vi "KN-OptionsToString.vi"(0 "Annulus IN":T2 {"End Angle" format="%.2f"; "Start Angle" format="%.2f"; "Center X" scale=0.0..1024.0}, 1 "Options IN":T5={"Search  Direction"=0, "Edge Options"={"Edge Polarity"=0, "Kernel Size"=13, "Width"=13, "Minimum Edge Strength"=52.0, "Interpolation Type"=enum."Bilinear Fixed", "Data Processing Method"=enum."Average"}} {"Search  Direction" items=["Outside to Inside", "Inside to Outside"]; "Edge Options"."Edge Polarity" items=["All Edges", "Rising Edges", "Falling Edges"]; "Edge Options"."Minimum Edge Strength" format="%.2f"; "Edge Options"."Width" step=2; "Edge Options"."Kernel Size" step=2}, 2 "Circle Fit Options":T1, 3 "(Color Threshold 1)":cluster{"Lower value":i32, "Upper value":i32}={"Lower value"=12, "Upper value"=253}) -> (14 "OptionsString Out":string=";1480.000;1115.000;378.000;757.000;0.000;0.000;0;1;3;3;10.000;4;0;1;1;1;1;65280;255;16776960;16711680;;3;10;3;23;255")   [LabVIEW 2015]
uses:
  <vilib>/vision/Measure.llb/Edge Options.ctl
  <vilib>/vision/Measure.llb/Edge Polarity.ctl
panel:
  out "Array":string[](array[string])
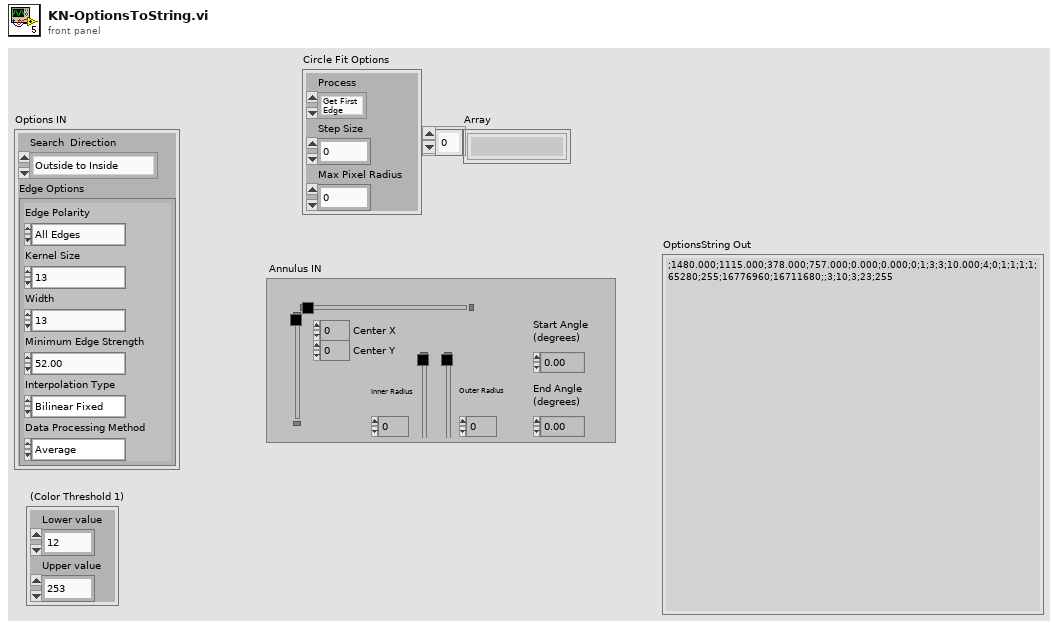
[diagram p1: front panel]
types:
  T1 = cluster{"Process":enum16{"Get First Edge", "Get First + Last Edge", "Get All Edges", "Get Best Edge"}, "Step Size":i32, "Max Pixel Radius":i32}
  T2 = typedef "IMAQ Circle" = cluster{"Center X":i32, "Center Y":i32, "Inner Radius":i32, "Outer Radius":i32, "Start Angle":dbl, "End Angle":dbl}
  T3 = typedef "Edge Options.ctl" = cluster{"Edge Polarity":T4, "Kernel Size":u32, "Width":u32, "Minimum Edge Strength":sgl, "Interpolation Type":enum32{"Zero Order", "Bilinear", "Quadratic", "Cubic", "Bilinear Fixed"}, "Data Processing Method":enum32{"Average", "Median"}}
  T4 = typedef "Edge Polarity.ctl" = u32
  T5 = cluster{"Search  Direction":u32, "Edge Options":T3}
  T6 = cluster{"Search  Direction":u32, "Edge Options":T3, "Show Search Area":bool, "Show Search Lines":bool, "Show Edges Found":bool, "Show Result":bool, "Search Area Color":u32, "Search Lines Color":u32, "Edge Locations Color":u32, "Result Color":u32, "Overlay Group Name":string}
  T7 = typedef "ROI Descriptor" = cluster{"Global Rectangle":i32[], "Contours":cluster{"ID":enum32{"External", "Internal"}, "Type":u32, "Coordinates":i32[]}[]}
  T8 = cluster{"ID":enum32{"External", "Internal"}, "Type":u32, "Coordinates":i32[]}[]
  T9 = cluster{"Lower value":string, "Upper value":string}
  T10 = cluster{"ID":enum32{"External", "Internal"}, "Type":u32, "Coordinates":i32[]}
  T11 = enum32{"Zero Order", "Bilinear", "Quadratic", "Cubic", "Bilinear Fixed"}
  T12 = cluster{"Process":string, "Step Size":string, "Max Pixel Radius":string}
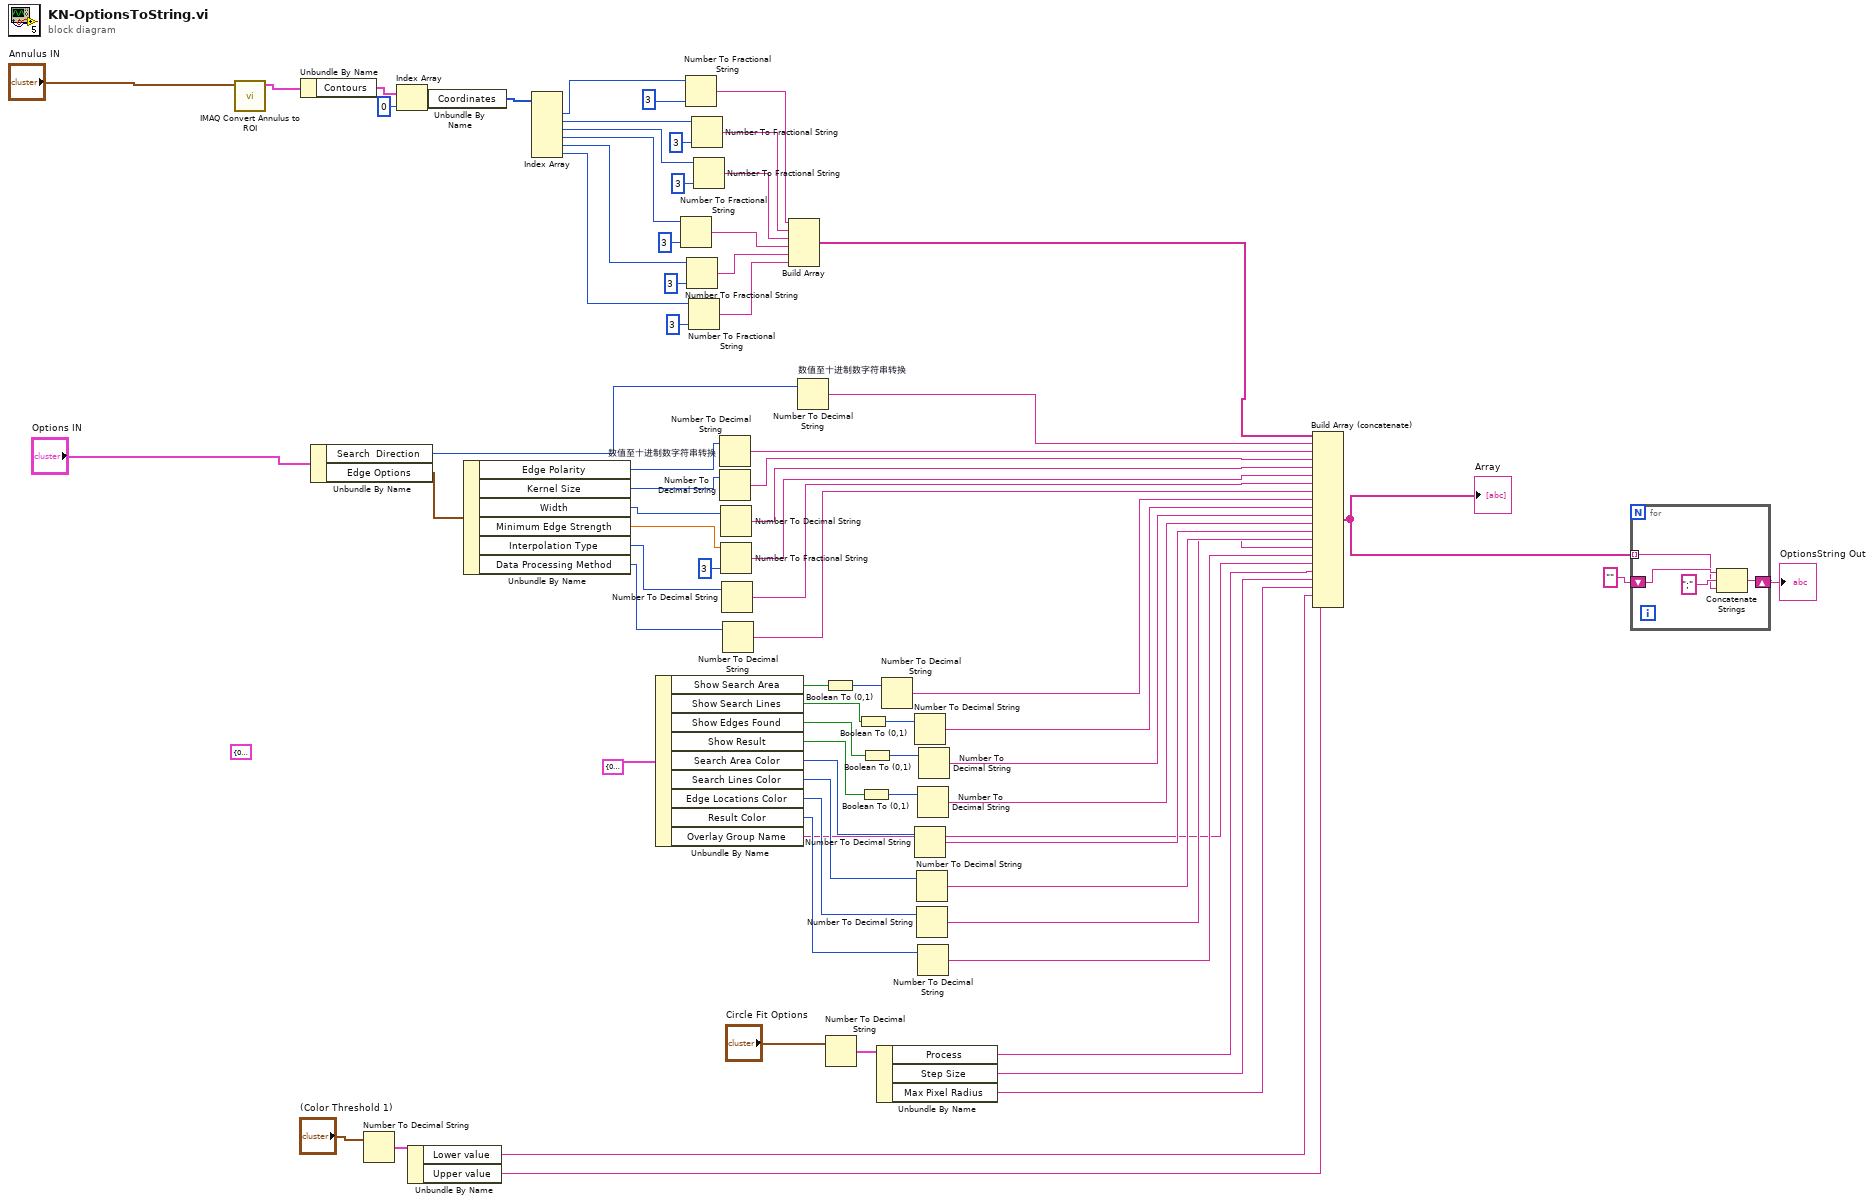
[diagram p0: block diagram]
diagram:
  (unwired) T6 {"Search  Direction"=0, "Edge Options"={"Edge Polarity"=0, "Kernel Size"=13, "Width"=13, "Minimum Edge Strength"=52.0, "Interpolation Type"=enum."Bilinear Fixed", "Data Processing Method"=enum."Average"}, "Show Search Area"=TRUE, "Show Search Lines"=FALSE, "Show Edges Found"=FALSE, "Show Result"=TRUE, "Search Area Color"=65280, "Search Lines Color"=255, "Edge Locations Color"=16776960, "Result Color"=16711680, "Overlay Group Name"=""} ("Options (Find Circular Edge 1)")
  n1 = call "IMAQ Convert Annulus to ROI"("Annulus"="Annulus IN") -> ("ROI Descriptor"=w29:T7)  [unwired: 8 in, 1 out]
  n2 = Unbundle By Name(w29) -> ("Contours"=w28:T8)
  n3 = Unbundle By Name("Options IN") -> ("Search  Direction"=w36:u32, "Edge Options"=w50:T3)
  n4 = Number To Decimal String(number="(Color Threshold 1)") -> (decimal integer string=w33:T9)  [unwired: 1 in]
  n5 = Index Array(array=w28, index=0 ("索引")) -> (element=w26:T10)
  n6 = Unbundle By Name(w33) -> ("Lower value"=w32:string, "Upper value"=w31:string)
  n7 = Unbundle By Name(w26) -> ("Coordinates"=w25:i32[])
  n8 = Unbundle By Name(w50) -> ("Edge Polarity"=w48:T4, "Kernel Size"=w47:u32, "Width"=w46:u32, "Minimum Edge Strength"=w45:sgl, "Interpolation Type"=w44:T11, "Data Processing Method"=w43:enum32{"Average", "Median"})
  n9 = Index Array(array=w25) -> (element #1=w24:i32, element #2=w17:i32, element #3=w16:i32, element #4=w15:i32, element #5=w14:i32, element #6=w13:i32)  [unwired: 6 in]
  n10 = Unbundle By Name(T6 {"Search  Direction"=0, "Edge Options"={"Edge Polarity"=0, "Kernel Size"=0, "Width"=0, "Minimum Edge Strength"=0.0, "Interpolation Type"=enum."Bilinear Fixed", "Data Processing Method"=enum."Average"}, "Show Search Area"=TRUE, "Show Search Lines"=FALSE, "Show Edges Found"=FALSE, "Show Result"=TRUE, "Search Area Color"=65280, "Search Lines Color"=255, "Edge Locations Color"=16776960, "Result Color"=16711680, "Overlay Group Name"=""} ("Options (Find Circular Edge 1)")) -> ("Show Search Area"=w74:bool, "Show Search Lines"=w69:bool, "Show Edges Found"=w68:bool, "Show Result"=w67:bool, "Search Area Color"=w66:u32, "Search Lines Color"=w65:u32, "Edge Locations Color"=w64:u32, "Result Color"=w63:u32, "Overlay Group Name"=w54:string)
  n11 = Number To Fractional String(number=w15, precision (6)=i16 3 ("精度(6)")) -> (F-format string=w9:string)  [unwired: 2 in]
  n12 = Number To Fractional String(number=w24, precision (6)=i16 3 ("精度(6)")) -> (F-format string=w12:string)  [unwired: 2 in]
  n13 = Number To Fractional String(number=w14, precision (6)=i16 3 ("精度(6)")) -> (F-format string=w8:string)  [unwired: 2 in]
  n14 = Number To Fractional String(number=w13, precision (6)=i16 3 ("精度(6)")) -> (F-format string=w7:string)  [unwired: 2 in]
  n15 = Number To Fractional String(number=w17, precision (6)=i16 3 ("精度(6)")) -> (F-format string=w11:string)  [unwired: 2 in]
  n16 = Number To Fractional String(number=w16, precision (6)=i16 3 ("精度(6)")) -> (F-format string=w10:string)  [unwired: 2 in]
  n17 = Number To Decimal String "数值至十进制数字符串转换"(number=w48) -> (decimal integer string=w42:string)  [unwired: 1 in]
  n18 = Number To Decimal String(number=w47) -> (decimal integer string=w41:string)  [unwired: 1 in]
  n19 = Number To Decimal String(number=w46) -> (decimal integer string=w40:string)  [unwired: 1 in]
  n20 = Number To Fractional String(number=w45, precision (6)=i16 3 ("精度(6)")) -> (F-format string=w39:string)  [unwired: 2 in]
  n21 = Number To Decimal String(number=w44) -> (decimal integer string=w38:string)  [unwired: 1 in]
  n22 = Number To Decimal String(number=w43) -> (decimal integer string=w37:string)  [unwired: 1 in]
  n23 = Build Array(w12, w11, w10, w9, w8, w7) -> (w6:string[])
  n24 = Number To Decimal String "数值至十进制数字符串转换"(number=w36) -> (decimal integer string=w35:string)  [unwired: 1 in]
  n25 = Boolean To (0,1)(Boolean=w74) -> (0, 1=w73:i16)
  n26 = Number To Decimal String(number="Circle Fit Options") -> (decimal integer string=w4:T12)  [unwired: 1 in]
  n27 = Boolean To (0,1)(Boolean=w69) -> (0, 1=w72:i16)
  n28 = Boolean To (0,1)(Boolean=w67) -> (0, 1=w70:i16)
  n29 = Boolean To (0,1)(Boolean=w68) -> (0, 1=w71:i16)
  n30 = Unbundle By Name(w4) -> ("Process"=w3:string, "Step Size"=w2:string, "Max Pixel Radius"=w1:string)
  n31 = Number To Decimal String(number=w73) -> (decimal integer string=w62:string)  [unwired: 1 in]
  n32 = Number To Decimal String(number=w72) -> (decimal integer string=w61:string)  [unwired: 1 in]
  n33 = Number To Decimal String(number=w66) -> (decimal integer string=w58:string)  [unwired: 1 in]
  n34 = Number To Decimal String(number=w65) -> (decimal integer string=w57:string)  [unwired: 1 in]
  n35 = Number To Decimal String(number=w64) -> (decimal integer string=w56:string)  [unwired: 1 in]
  n36 = Number To Decimal String(number=w70) -> (decimal integer string=w59:string)  [unwired: 1 in]
  n37 = Number To Decimal String(number=w63) -> (decimal integer string=w55:string)  [unwired: 1 in]
  n38 = Number To Decimal String(number=w71) -> (decimal integer string=w60:string)  [unwired: 1 in]
  n39 = Build Array (concatenate)(w6, w35, w42, w41, w40, w39, w38, w37, w62, w61, w60, w59, w58, w57, w56, w55, w54, w3, w2, w1, w32, w31) -> (w52:string[])
  "Array" <- w52
  n40 = for {
    tunnel: w52 -> [w77] mode=indexing
    shift-right: [w80] -> w51
    shift-left: "" -> [w78]
    n41 = Concatenate Strings(w78, ";" ("字符串"), w77) -> (w80:string)
  }
  "OptionsString Out" <- w51
